vi "UpdateStepIndex.vi"(8 "error in (no error)":errorcluster, 11 "Index":T1) -> (0 "error out":errorcluster)   [LabVIEW 2016, in "SeqProcessor.lvlib"]
uses:
  SeqProcessor.lvlib
  controls/StepIndex.ctl
  <vilib>/addons/PointValueMap/subVIs/Point_Write_variant.vi
  <vilib>/addons/PointValueMap/PointValueMap.lvlib
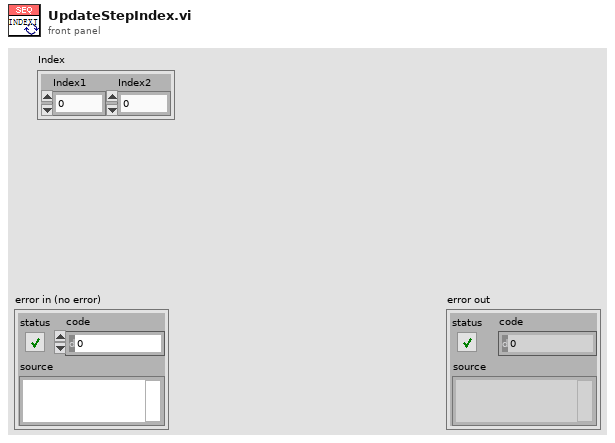
[diagram p1: front panel]
types:
  T1 = typedef "SeqProcessor.lvlib/StepIndex.ctl" = cluster{"Index1":u32, "Index2":u32}
  T2 = typedef "PointValueMap.lvlib/PointMap.ctl" = refnum<data-value>
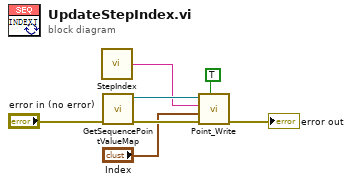
[diagram p0: block diagram]
diagram:
  n1 = call "StepIndex.vi"() -> ("StepIndex"=w1:string)  [unwired: 5 in]
  n2 = call "GetSequencePointValueMap.vi"("error in (no error)"="error in (no error)") -> ("error out"=w6:errorcluster, "SeqMap"=w5:T2)  [unwired: 9 in]
  n3 = call-poly <vilib>:"Point_Write.vi"("Auto Create?"=TRUE, "Error In"=w6, "Value"="Index", "Tag"=w1, "Map"=w5) -> ("Error Out"=→"error out":errorcluster)  [unwired: 5 in, 1 out]
